vi "Search_for_Product.vi"(8 "error in (no error)":errorcluster, 10 "Search Number, Name or Producer":string, 11 "Products":T1[](array[typedef])) -> (0 "error out":errorcluster, 3 "Product Index":i32)   [LabVIEW 2020]
doc: "This VI search for element <b>search</b> in <b>array of #typedef Products</b> and returns the index of founded element. If any elements does not match the search expression then program returns index -1."
uses:
  #typedef_Product.ctl
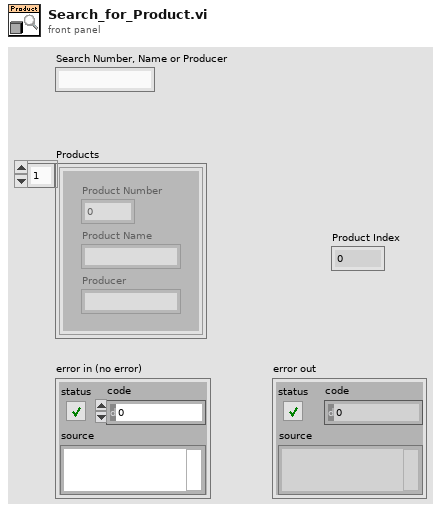
[diagram p1: front panel]
types:
  T1 = typedef "#typedef_Product.ctl" = cluster{"Product Number":i32, "Product Name":string, "Producer":string}
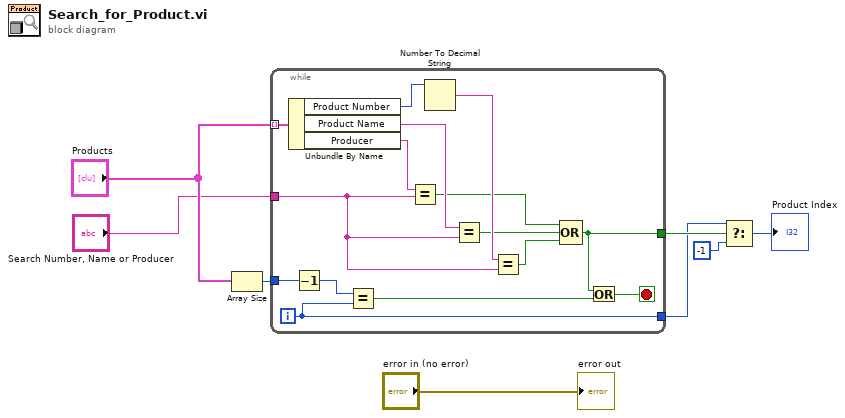
[diagram p0: block diagram]
diagram:
  n1 = Array Size(array="Products") -> (size(s)=w8:i32)
  n2 = while {
    tunnel: "Products" -> [w15] mode=indexing
    tunnel: "Search Number, Name or Producer" -> [w20]
    tunnel: w8 -> [w14]
    tunnel: [w13] -> w3
    tunnel: [w9] -> w4
    i -> [w13]
    stop <- w11 stop-if-true
    n3 = Unbundle By Name(w15) -> ("Product Number"=w23:i32, "Product Name"=w21:string, "Producer"=w22:string)
    n4 = Decrement(x=w14) -> (x-1=w12:i32)
    n5 = Equal?(x=w12, y=w13) -> (x = y?=w10:bool)
    n6 = Equal?(x=w22, y=w20) -> (x = y?=w18:bool)
    n7 = Number To Decimal String(number=w23) -> (decimal integer string=w19:string)  [unwired: 1 in]
    n8 = Equal?(x=w21, y=w20) -> (x = y?=w17:bool)
    n9 = Equal?(x=w19, y=w20) -> (x = y?=w16:bool)
    n10 = Compound Arithmetic op=OR(w18, w17, w16) -> (w9:bool)
    n11 = Or(x=w9, y=w10) -> (x .or. y?=w11:bool)
  }
  n12 = Select(t=w3, s=w4, f=-1) -> (s? t:f=→"Product Index":i32)
  "error out" <- "error in (no error)"
